vi "Table-Delete empty rows at the end.vi"(11 "Value in":string[][](array[string])) -> (3 "Value out":string[][](array[string]))   [LabVIEW 2020]
uses:
  <userlib>/_OpenG.lib/array/array.llb/Search 1D Array (String)__ogtk.vi
  <userlib>/_OpenG.lib/array/array.llb/Delete Elements from 1D Array (String)__ogtk.vi
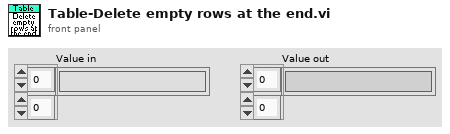
[diagram p1: front panel]
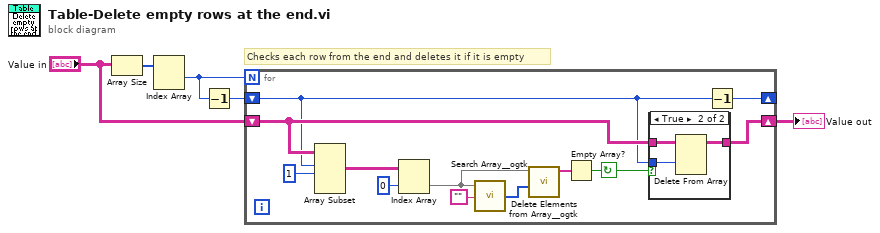
[diagram p0: block diagram]
diagram:
  # "Checks each row from the end and deletes it if it is empty"
  n1 = Array Size(array="Value in") -> (size(s)=w2:i32[])
  n2 = Index Array(array=w2) -> (element #1=w4:i32)  [unwired: 2 in, 1 out]
  n3 = Decrement(x=w4) -> (x-1=w3:i32)
  n4 = for {
    N: w4 -> [_]
    shift-right: [w17] -> _
    shift-left: w3 -> [w6]
    shift-right: [w9] -> w5
    shift-left: "Value in" -> [w8]
    stop <- w7 continue-if-true
    n5 = Array Subset "Array Subset"(array=w8, index (row)=w6, length (row)=1 ("length")) -> (w15:string[][])  [unwired: 2 in]
    n6 = Index Array "Index Array"(array=w15, index (row)=0) -> (element=w11:string[])  [unwired: 1 in]
    n7 = call-poly <userlib>:"Search Array__ogtk.vi"("Array"=w11, "Element Data"="") -> ("Indices of Elements"=w12:i32[])  [unwired: 7 in]
    n8 = call-poly <userlib>:"Delete Elements from Array__ogtk.vi"("indices"=w12, "array"=w11) -> ("array w/ subset deleted"=w10:string[])  [unwired: 8 in, 1 out]
    n9 = Empty Array?(array=w10) -> (empty?=w7:bool)
    n10 = case shown="True" w7 {
      tunnel: w8 -> [w18 w21]
      tunnel: [w18 w20] -> w9
      tunnel: w6 -> [_ w19]
      frame False {
      }
      frame True {
        n11 = Delete From Array(array=w21, index (row)=w19) -> (array with subset deleted=w20:string[][])  [unwired: 2 in, 1 out]
      }
    }
    n12 = Decrement(x=w6) -> (x-1=w17:i32)
  }
  "Value out" <- w5
